vi "rp_align_objects_dialog.vi"(8 "error in (no error)":errorcluster) -> (0 "error out":errorcluster, 3 "align out":T1(ring))   [LabVIEW 2019]
uses:
  <vilib>/event_ctls.llb/eventvkey.ctl
panel:
  in  "v_compress":bool
  out "VKey":T2
  out "Char":i16
  in  "right":bool
  in  "left":bool
  in  "bottom":bool
  in  "top":bool
  # "Press Up, Down, Left, Right, X or Esc"
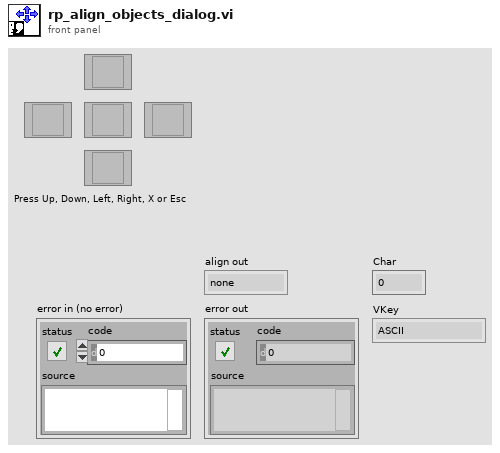
[diagram p1: front panel]
types:
  T1 = enum32{"none", "top", "bottom", "left", "right", "v_compress"}
  T2 = typedef "eventvkey.ctl" = enum16{"ASCII", "Enter", "Return", "Shift", "Ctrl", "Alt", "Cmd", "Opt", "Caps", "NumLock", "Clear", "Break", "Up", "Down", "Left", "Right", "Insert", "Delete", "Home", "End", "PageUp", "PageDown", "Escape", "Help", "Pause", "ScrollLock", "F1", "F2", "F3", "F4", "F5", "F6", "F7", "F8", "F9", "F10", "F11", "F12", "F13", "F14", "F15", "F16", "F17", "F18", "F19", "F20", "F21", "F22", "F23", "F24", "Play", "VolumeUp", "VolumeDown", "Mute", "Two Byte Char"}
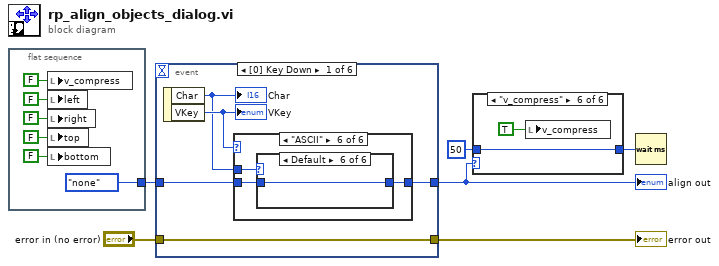
[diagram p0: block diagram]
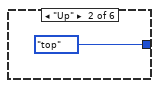
[diagram p3: hidden frame]
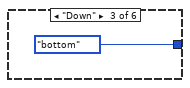
[diagram p4: hidden frame]
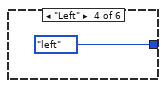
[diagram p5: hidden frame]
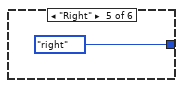
[diagram p6: hidden frame]
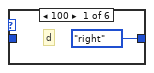
[diagram p7: hidden frame]
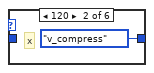
[diagram p8: hidden frame]
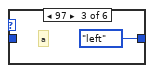
[diagram p9: hidden frame]
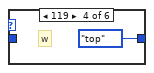
[diagram p10: hidden frame]
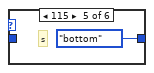
[diagram p11: hidden frame]
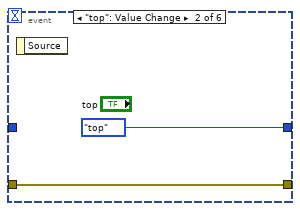
[diagram p12: hidden frame]
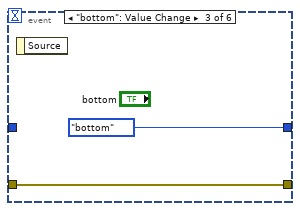
[diagram p13: hidden frame]
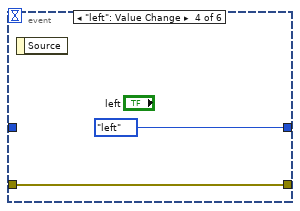
[diagram p14: hidden frame]
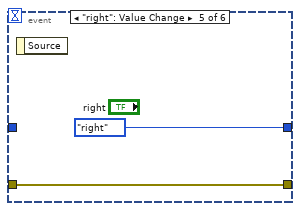
[diagram p15: hidden frame]
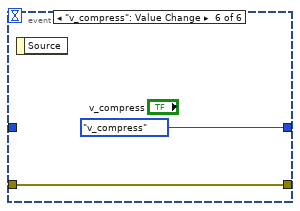
[diagram p16: hidden frame]
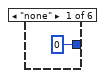
[diagram p17: hidden frame]
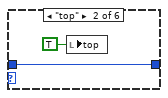
[diagram p18: hidden frame]
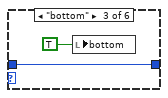
[diagram p19: hidden frame]
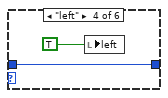
[diagram p20: hidden frame]
diagram:
  n1 = flat-sequence {
    tunnel: [T1."none" ("default align")] -> w4
    frame #0 {
      n2 = local write "v_compress"(FALSE ("distribute")) -> ()
      n3 = local write "left"(FALSE ("left")) -> ()
      n4 = local write "right"(FALSE ("right")) -> ()
      n5 = local write "top"(FALSE ("top")) -> ()
      n6 = local write "bottom"(FALSE ("bottom")) -> ()
    }
  }
  n7 = event shown="[0] Key Down" {
    selector: _ -> [_ _ _ _ _ _]
    dyn-events: _ -> [_ _ _ _ _ _]
    timeout: _ -> [_ _ _ _ _ _]
    tunnel: [w14 T1."top" ("default align") T1."bottom" ("default align") T1."left" ("default align") T1."right" ("default align") T1."v_compress" ("default align")] -> w3
    tunnel: "error in (no error)" -> [w17 w33 w35 w37 w39 w41]
    tunnel: [w17 w33 w35 w37 w39 w41] -> w5
    tunnel: w4 -> [w15 _ _ _ _ _]
    event Key Down {
      n8 = event-data() -> ("Char"=w13:i16, "VKey"=w16:T2)  [unwired: 1 in]
      "Char" <- w13
      "VKey" <- w16
      n9 = case shown="\"ASCII\"" w16 {
        tunnel: [w18 T1."top" ("default align") T1."bottom" ("default align") T1."left" ("default align") T1."right" ("default align") w24] -> w14
        tunnel: w15 -> [w18 _ _ _ _ w23]
        tunnel: w13 -> [_ _ _ _ _ w25]
        frame "Escape", Default {
        }
        frame "Up" {
        }
        frame "Down" {
        }
        frame "Left" {
        }
        frame "Right" {
        }
        frame "ASCII" {
          n10 = case shown="Default" w25 {
            tunnel: [T1."right" ("default align") T1."v_compress" ("default align") T1."left" ("default align") T1."top" ("default align") T1."bottom" ("default align") w31] -> w24
            tunnel: w23 -> [_ _ _ _ _ w31]
            frame 100 {
              # "d"
            }
            frame 120 {
              # "x"
            }
            frame 97 {
              # "a"
            }
            frame 119 {
              # "w"
            }
            frame 115 {
              # "s"
            }
            frame Default {
            }
          }
        }
      }
    }
    event "top": Value Change {
      n11 = event-data() -> ()  [unwired: 1 in, 1 out]
    }
    event "bottom": Value Change {
      n12 = event-data() -> ()  [unwired: 1 in, 1 out]
    }
    event "left": Value Change {
      n13 = event-data() -> ()  [unwired: 1 in, 1 out]
    }
    event "right": Value Change {
      n14 = event-data() -> ()  [unwired: 1 in, 1 out]
    }
    event "v_compress": Value Change {
      n15 = event-data() -> ()  [unwired: 1 in, 1 out]
    }
  }
  "align out" <- w3
  "error out" <- w5
  n16 = case shown="\"v_compress\"" w3 {
    tunnel: [u32 0 ("milliseconds to wait") w44 w46 w48 w50 w52] -> w1
    tunnel: u32 50 ("milliseconds to wait") -> [_ w44 w46 w48 w50 w52]
    frame "none" {
    }
    frame "top" {
      n17 = local write "top"(TRUE ("top")) -> ()
    }
    frame "bottom" {
      n18 = local write "bottom"(TRUE ("top")) -> ()
    }
    frame "left" {
      n19 = local write "left"(TRUE ("top")) -> ()
    }
    frame "right" {
      n20 = local write "right"(TRUE ("top")) -> ()
    }
    frame "v_compress" {
      n21 = local write "v_compress"(TRUE ("top")) -> ()
    }
  }
  n22 = Wait (ms)(milliseconds to wait=w1) -> ()  [unwired: 1 out]
